vi "Close Test Group Manager.vi"(8 "error in (no error)":errorcluster, 11 "QPA Measurement in":refnum<class "QPA Measurement.lvclass">) -> (0 "error out":errorcluster, 3 "QPA Measurement out":refnum<class "QPA Measurement.lvclass">)   [LabVIEW 2016, in "QPA Measurement.lvlib" / "QPA Measurement.lvclass"]
uses:
  QPA Measurement.lvclass
  QPA Measurement.lvclass/QPA Measurement.ctl
  Plugins/Test Group Manager.lvlibp/Test Group Manager.lvclass
  Protected Methods/Read Test Group Manager.vi
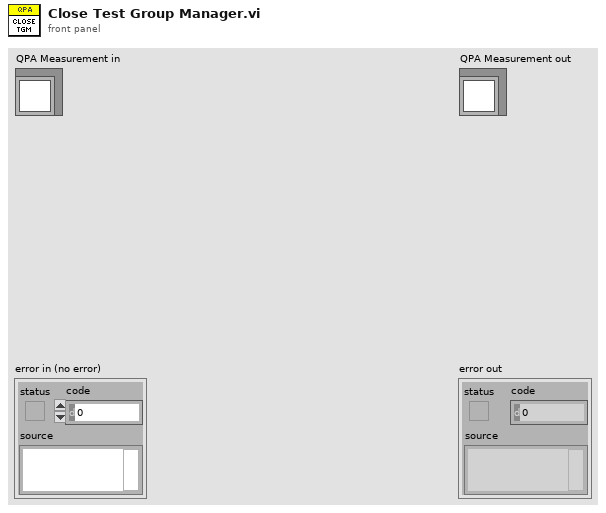
[diagram p1: front panel]
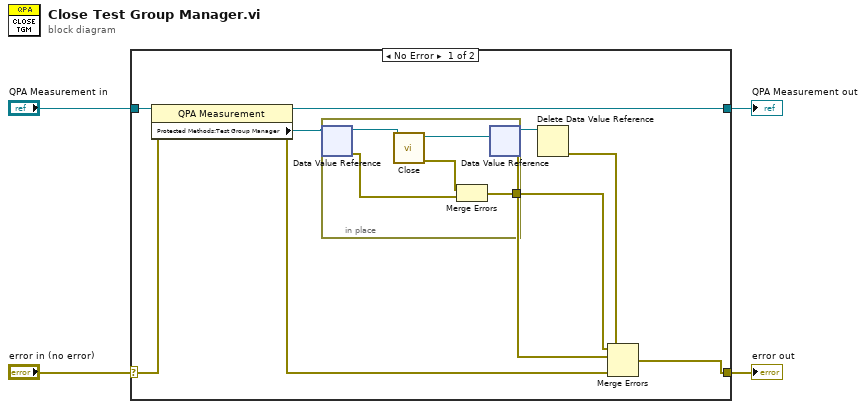
[diagram p0: block diagram]
diagram:
  n1 = case shown="No Error" "error in (no error)" {
    selector: "error in (no error)" -> [w14 w21]
    tunnel: [w5 w21] -> w3
    tunnel: [w12 w20] -> w1
    tunnel: "QPA Measurement in" -> [w13 w20]
    frame No Error {
      n2 = property class="QPA Measurement"(reference=w13, error in=w14) -> (reference out=w12:refnum<class "QPA Measurement.lvclass">, error out=w6:errorcluster, "Protected Methods:Test Group Manager"=w11:refnum<data-value>)
      n3 = in-place {
        in-place-border: [w15] -> w9
        n4 = in-place-dvr #1(w11) -> (w19:refnum<class "Test Group Manager.lvclass">, w16:errorcluster)
        n5 = call "Close.vi"("Test Group Manager in"=w19) -> ("error out"=w17:errorcluster, "Test Group Manager out"=w18:refnum<class "Test Group Manager.lvclass">)  [unwired: 9 in]
        n6 = Merge Errors(w17, w16) -> (w15:errorcluster)
        n7 = in-place-dvr #1(w18) -> (w10:refnum<data-value>, w8:errorcluster)
      }
      n8 = Delete Data Value Reference(data value reference=w10) -> (error out=w7:errorcluster)  [unwired: 1 in, 1 out]
      n9 = Merge Errors(w9, w8, w7, w6) -> (w5:errorcluster)
    }
    frame Error {
    }
  }
  "error out" <- w3
  "QPA Measurement out" <- w1
